vi "Motor control template.vi"() -> ()   [LabVIEW 2020]
uses:
  <vilib>/DAQmx/configure/timing.llb/DAQmx Timing (Implicit).vi
  <vilib>/DAQmx/create/channels.llb/DAQmx Create Channel (CO-Pulse Generation-Frequency).vi
  <vilib>/Utility/error.llb/DialogType.ctl
  <resource>/objmgr/daqmx.rc
  <vilib>/DAQmx/write.llb/DAQmx Write (Counter Frequency 1Chan 1Samp).vi
  Risley Driver Main.vit
panel:
  out "Numeric Control":i32
  in  "Error In 2":errorcluster
  in  "Error In":errorcluster
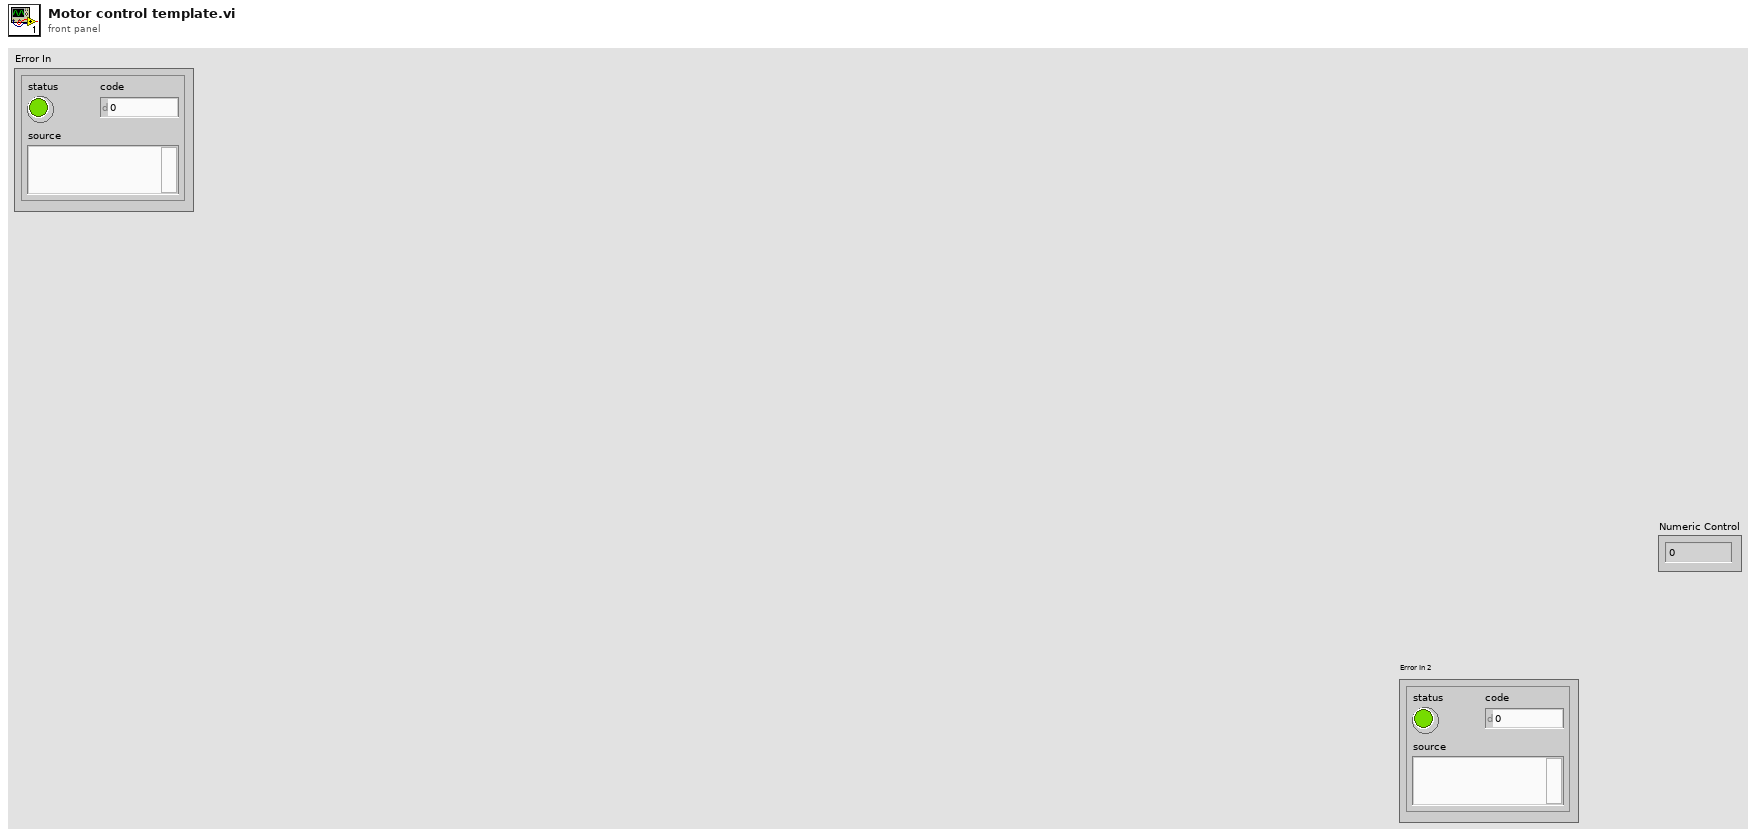
[diagram p1: front panel]
types:
  T1 = enum16{"Starting", "Ramp Up", "Idle", "Ramp Down", "Stopping", "Step and Dwell"}
  T2 = typedef "DialogType.ctl" = u16
  T3 = enum16{"Starting", "Ramp Up", "Idle", "Ramp Down", "Stopping"}
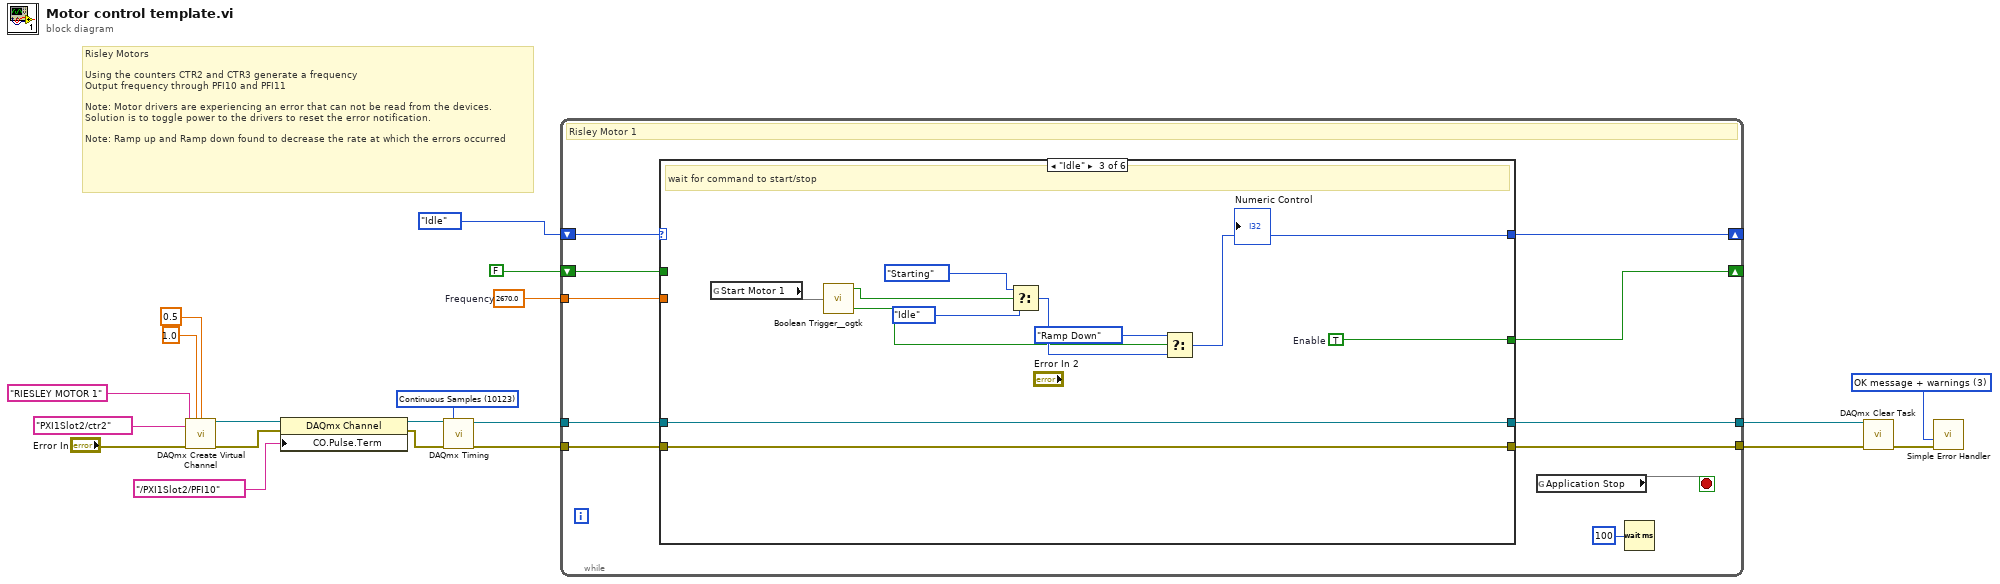
[diagram p0: block diagram]
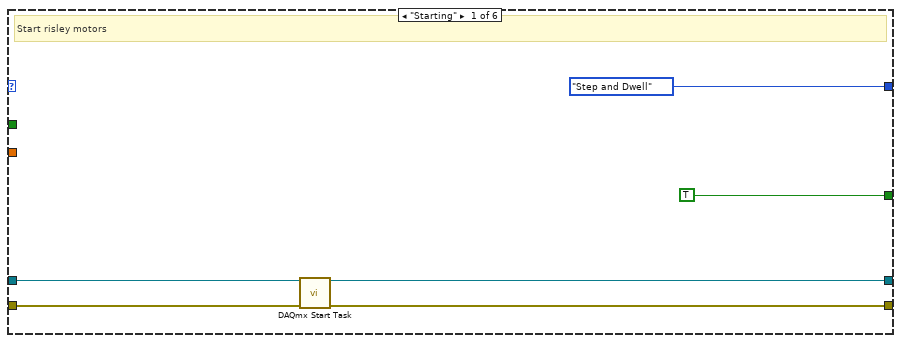
[diagram p2: hidden frame]
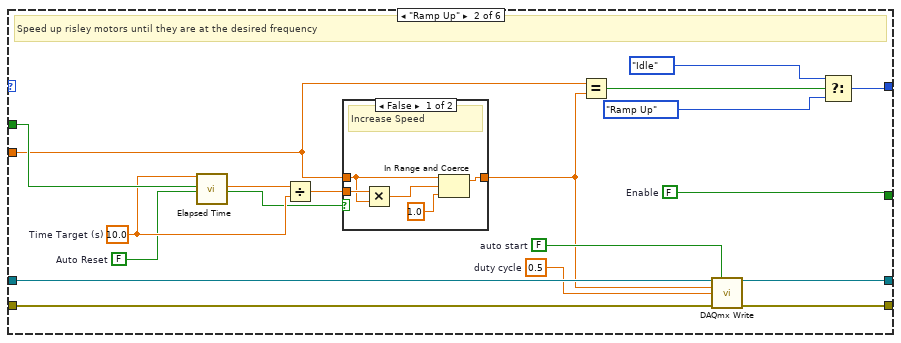
[diagram p3: hidden frame]
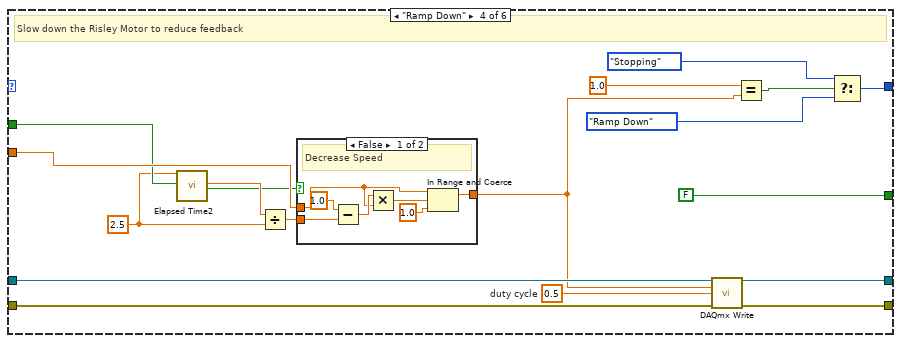
[diagram p5: hidden frame]
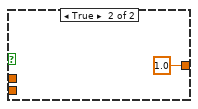
[diagram p6: hidden frame]
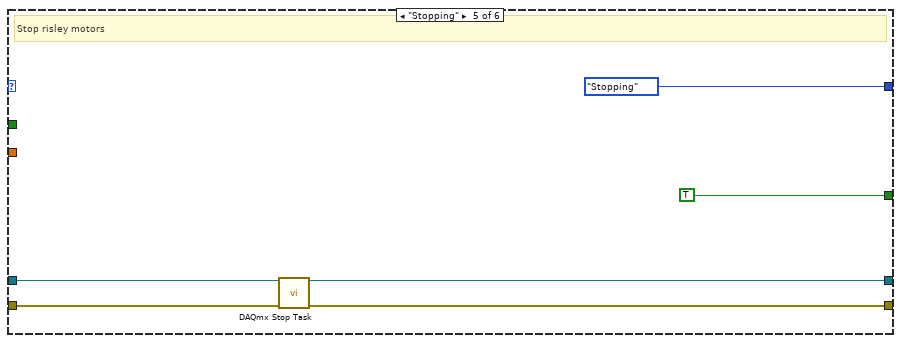
[diagram p7: hidden frame]
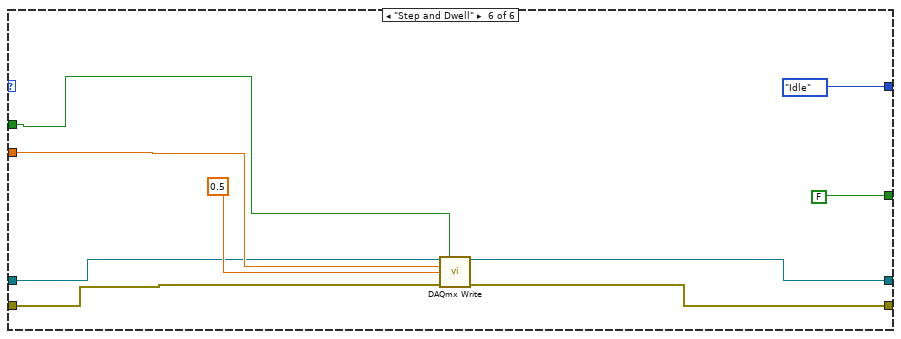
[diagram p8: hidden frame]
diagram:
  w7 = 2670.0  # Frequency
  w17 = T2 3 items=["no dialog", "OK message", "continue or stop message", "OK message + warnings", "continue/stop + warnings"] ("type of dialog (OK msg:1)")
  w19 = 10123 items=["Finite Samples"=10178, "Continuous Samples"=10123] ("sample mode")
  # "Risley Motors\n\nUsing the counters CTR2 and CTR3 generate a frequency\nOutput frequency through PFI10 and PFI11\n\nNote: Motor drivers are experiencing an error that can not be read from the devices. \nSolution is to toggle power to the drivers to reset the error notification. \n\nNote: Ramp up and Ramp down found to decrease the rate at which the errors occurred"
  n1 = call-poly <vilib>:"DAQmx Create Virtual Channel.vi"("frequency"=1.0, "duty cycle"=0.5, "counter"=tag "PXI1Slot2/ctr2" ("Counter(s)"), "name to assign"="RIESLEY MOTOR 1", "error in"="Error In") -> ("task out"=w16:refnum<k21>, "error out"=w13:errorcluster)  [unwired: 9 in]
  n2 = property class="DAQmx Channel"(reference=w16, error in=w13, "CO.Pulse.Term"=tag "/PXI1Slot2/PFI10") -> (reference out=w15:refnum<k21>, error out=w14:errorcluster)
  n3 = call-poly <vilib>:"DAQmx Timing.vi"("task/channels in"=w15, "sample mode"=w19, "error in"=w14) -> ("task out"=w5:refnum<k21>, "error out"=w4:errorcluster)  [unwired: 11 in]
  n4 = while {
    shift-right: [w28] -> _
    shift-left: T1."Idle" -> [w31]
    tunnel: w4 -> [w27]
    tunnel: w7 -> [w26]
    shift-right: [w24] -> _
    shift-left: FALSE ("Enable") -> [w25]
    tunnel: w5 -> [w29]
    tunnel: [w30] -> w9
    tunnel: [w22] -> w2
    stop <- w21 stop-if-true
    # "Risley Motor 1"
    n5 = case shown="\"Idle\"" w31 {
      tunnel: [w32 w47 w71 w91 w103 w107] -> w30
      tunnel: w29 -> [w37 w56 w71 w90 w104 w106]
      tunnel: [T1."Step and Dwell" ("f") w53 w66 w85 T3."Stopping" ("f") T1."Idle" ("f")] -> w28
      tunnel: w27 -> [w36 w55 w70 w89 w105 w109]
      tunnel: [w33 w46 w70 w88 w102 w111] -> w22
      tunnel: w26 -> [_ w38 _ w86 _ w110]
      tunnel: w25 -> [_ w50 _ w79 _ w112]
      tunnel: [TRUE ("Enable") w49 w69 FALSE ("Enable") TRUE ("Enable") FALSE] -> w24
      frame "Starting" {
        # "Start risley motors"
        n6 = call <vilib>:"DAQmx Start Task.vi"("task/channels in"=w37, "error in"=w36) -> ("task out"=w32:refnum<k21>, "error out"=w33:errorcluster)  [unwired: 12 in]
      }
      frame "Ramp Up" {
        w39 = FALSE  # Auto Reset
        w42 = 10.0  # Time Target (s)
        w45 = FALSE  # auto start
        w49 = FALSE  # Enable
        w54 = 0.5  # duty cycle
        # "Speed up risley motors until they are at the desired frequency"
        n7 = call "Elapsed Time"("Time Target (s)"=w42, "Reset"=w50, "Auto Reset"=w39) -> ("Elapsed Time (s)"=w43:dbl, "Time has Elapsed"=w40:bool)  [unwired: 9 in, 6 out]
        n8 = Divide(x=w43, y=w42) -> (x/y=w41:dbl)
        n9 = case shown="False" w40 {
          tunnel: w41 -> [w61 _]
          tunnel: w38 -> [w59 w62]
          tunnel: [w57 w62] -> w44
          frame False {
            # "Increase Speed"
            n10 = Multiply(x=w61, y=w59) -> (x*y=w60:dbl)
            n11 = In Range and Coerce(upper limit=w59, x=w60, lower limit=1.0) -> (coerced(x)=w57:dbl)  [unwired: 1 out]
          }
          frame True {
          }
        }
        n12 = Equal?(x=w38, y=w44) -> (x = y?=w48:bool)
        n13 = call-poly <vilib>:"DAQmx Write.vi"("task/channels in"=w56, "auto start"=w45, "frequency"=w44, "duty cycle"=w54, "error in"=w55) -> ("task out"=w47:refnum<k21>, "error out"=w46:errorcluster)  [unwired: 8 in, 1 out]
        n14 = Select(t=T3."Idle", s=w48, f=T3."Ramp Up") -> (s? t:f=w53:T3)
      }
      frame "Idle" {
        w69 = TRUE  # Enable
        # "wait for command to start/stop"
        n15 = global read "Risley Driver Main.vit" "Start Motor 1"() -> (w63)
        n16 = call <userlib>:"Boolean Trigger__ogtk.vi"("Boolean Input"=w63) -> ("Rising Edge"=w68:bool, "Falling Edge"=w64:bool)  [unwired: 1 in]
        n17 = Select(t=T1."Starting", s=w68, f=T1."Idle") -> (s? t:f=w65:T1)
        n18 = Select(t=T1."Ramp Down", s=w64, f=w65) -> (s? t:f=w66:T1)
      }
      frame "Ramp Down" {
        w76 = 2.5 ("Time Target (s)")
        w87 = 0.5  # duty cycle
        # "Slow down the Risley Motor to reduce feedback"
        n19 = call "Elapsed Time2"("Time Target (s)"=w76, "Reset"=w79) -> ("Elapsed Time (s)"=w77:dbl, "Time has Elapsed"=w74:bool)  [unwired: 10 in, 6 out]
        n20 = Divide(x=w77, y=w76) -> (x/y=w75:dbl)
        n21 = case shown="False" w74 {
          tunnel: [w93 1.0] -> w78
          tunnel: w86 -> [w92 _]
          tunnel: w75 -> [w98 _]
          frame False {
            # "Decrease Speed"
            n22 = Subtract(x=1.0, y=w98) -> (x-y=w96:dbl)
            n23 = Multiply(x=w96, y=w92) -> (x*y=w94:dbl)
            n24 = In Range and Coerce(upper limit=w92, x=w94, lower limit=1.0) -> (coerced(x)=w93:dbl)  [unwired: 1 out]
          }
          frame True {
          }
        }
        n25 = call-poly <vilib>:"DAQmx Write.vi"("task/channels in"=w90, "frequency"=w78, "duty cycle"=w87, "error in"=w89) -> ("task out"=w91:refnum<k21>, "error out"=w88:errorcluster)  [unwired: 9 in, 1 out]
        n26 = Equal?(x=1.0, y=w78) -> (x = y?=w80:bool)
        n27 = Select(t=T3."Stopping", s=w80, f=T3."Ramp Down") -> (s? t:f=w85:T3)
      }
      frame "Stopping" {
        # "Stop risley motors"
        n28 = call <vilib>:"DAQmx Stop Task.vi"("task/channels in"=w104, "error in"=w105) -> ("task out"=w103:refnum<k21>, "error out"=w102:errorcluster)  [unwired: 12 in]
      }
      frame "Step and Dwell" {
        n29 = call-poly <vilib>:"DAQmx Write.vi"("task/channels in"=w106, "auto start"=w112, "frequency"=w110, "duty cycle"=0.5, "error in"=w109) -> ("task out"=w107:refnum<k21>, "error out"=w111:errorcluster)  [unwired: 8 in, 1 out]
      }
    }
    n30 = global read "Risley Driver Main.vit" "Application Stop"() -> (w21)
    n31 = Wait (ms)(milliseconds to wait=u32 100) -> ()  [unwired: 1 out]
  }
  n32 = call <vilib>:"DAQmx Clear Task.vi"("task in"=w9, "error in"=w2) -> ("error out"=w20:errorcluster)  [unwired: 13 in]
  n33 = call <vilib>:"Simple Error Handler.vi"("type of dialog (OK msg:1)"=w17, "error in (no error)"=w20) -> ()  [unwired: 3 in, 5 out]
